vi "save parameters.vi"   [LabVIEW 2014]
uses:
  Start all VIs Globals.vi
  TIRF Lock/autofocus-globals.vi
  <vilib>/Utility/config.llb/Write Key (Boolean).vi
  <vilib>/Utility/config.llb/Write Key (Double).vi
  <vilib>/Utility/config.llb/Write Key (I32).vi
  <vilib>/Utility/config.llb/Write Key (U32).vi
  <vilib>/Utility/config.llb/NI_LVConfig.lvlib
types:
  T1 = enum32{"Invalid", "Standard", "Closed", "Hidden", "Minimized", "Maximized"}
  T2 = typedef "NI_LVConfig.lvlib/Config Data RefNum.ctl" = refnum<k1>
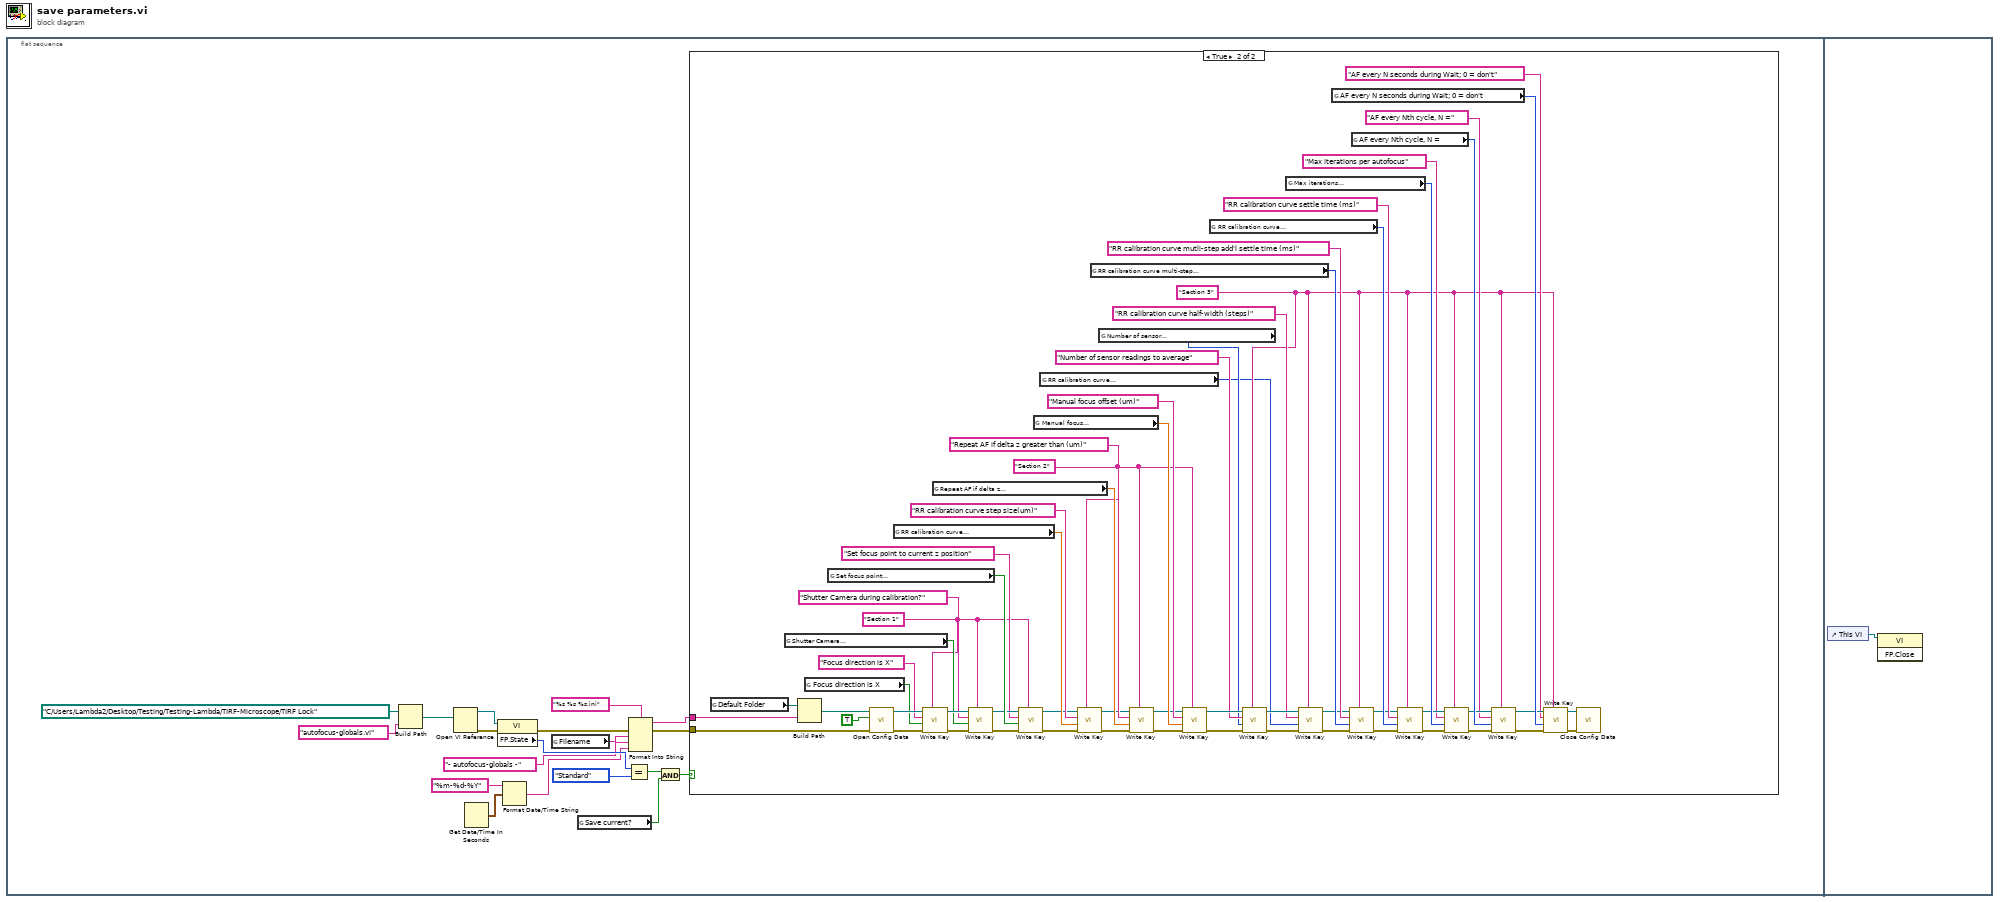
[diagram p0: block diagram]
diagram:
  n1 = flat-sequence {
    frame #0 {
      n2 = Build Path(base path=path "C:/Users/Lambda2/Desktop/Testing/Testing-Lambda/TIRF-Microscope/TIRF Lock", name or relative path="autofocus-globals.vi") -> (appended path=w18:path)
      n3 = Open VI Reference(vi path=w18) -> (vi reference=w17:refnum<vi>, error out=w16:errorcluster)  [unwired: 1 in, 4 out]
      n4 = Get Date/Time In Seconds() -> (seconds since 1Jan1904=w1:timestamp)
      n5 = property class="VI"(reference=w17, error in=w16) -> (error out=w7:errorcluster, "FP.State"=w13:T1)  [unwired: 1 out]
      n6 = Format Date/Time String(time format string (%c)="%m-%d-%Y", seconds (now)=w1) -> (date/time string=w3:string)  [unwired: 1 in]
      n7 = global read "Start all VIs Globals.vi" "Filename"() -> (w4:string)
      n8 = global read "Start all VIs Globals.vi" "Save current?"() -> (w10:bool)
      n9 = Equal?(x=w13, y=T1."Standard") -> (x = y?=w12:bool)
      n10 = Format Into String(format string="%s %s %s.ini", error in=w7, w4, "- autofocus-globals -", w3) -> (resulting string=w8:string, error out=w6:errorcluster)  [unwired: 1 in]
      n11 = And(x=w12, y=w10) -> (x .and. y?=w11:bool)
      n12 = case shown="True" w11 {
        tunnel: w6 -> [_ w32]
        tunnel: w8 -> [_ w34]
        frame False {
        }
        frame True {
          w22 = "Section 3"
          w38 = "Section 2"
          w39 = "Section 1"
          n13 = global read "Start all VIs Globals.vi" "Default Folder"() -> (w35:path)
          n14 = global read "autofocus-globals.vi" "Shutter Camera\nduring calibration?"() -> (w72:bool)
          n15 = Build Path(base path=w35, name or relative path=w34) -> (appended path=w33:path)
          n16 = global read "autofocus-globals.vi" "Focus direction is X"() -> (w78:bool)
          n17 = global read "autofocus-globals.vi" "Set focus point\nto current z position"() -> (w71:bool)
          n18 = call <vilib>:"Open Config Data.vi"("error in (no error)"=w32, "create file if necessary (T)"=TRUE, "configuration file path"=w33) -> ("error out"=w80:errorcluster, "refnum"=w79:T2)  [unwired: 7 out]
          n19 = global read "autofocus-globals.vi" "RR calibration curve\nstep size (um)"() -> (w68:ext)
          n20 = call-poly <vilib>:"Write Key.vi"("section"=w39, "error in (no error)"=w80, "value"=w78, "key"="Focus direction is X", "refnum"=w79) -> ("error out"=w76:errorcluster, "refnum out"=w74:T2)  [unwired: 5 out]
          n21 = global read "autofocus-globals.vi" "Repeat AF if delta z \ngreater than (um)"() -> (w66:dbl)
          n22 = call-poly <vilib>:"Write Key.vi"("section"=w39, "error in (no error)"=w76, "value"=w72, "key"="Shutter Camera during calibration?", "refnum"=w74) -> ("error out"=w75:errorcluster, "refnum out"=w70:T2)  [unwired: 5 out]
          n23 = call-poly <vilib>:"Write Key.vi"("section"=w39, "error in (no error)"=w75, "value"=w71, "key"="Set focus point to current z position", "refnum"=w70) -> ("error out"=w67:errorcluster, "refnum out"=w59:T2)  [unwired: 5 out]
          n24 = global read "autofocus-globals.vi" "Manual focus\noffset (um)"() -> (w65:dbl)
          n25 = global read "autofocus-globals.vi" "RR calibration curve\nhalf-width  (steps)"() -> (w20:u32)
          n26 = call-poly <vilib>:"Write Key.vi"("section"=w38, "error in (no error)"=w67, "value"=w68, "key"="RR calibration curve step size(um)", "refnum"=w59) -> ("error out"=w64:errorcluster, "refnum out"=w58:T2)  [unwired: 3 in, 2 out]
          n27 = global read "autofocus-globals.vi" "RR calibration curve multi-step\nadd'l settle time (ms)"() -> (w26:u16)
          n28 = global read "autofocus-globals.vi" "Number of sensor\nreadings to average"() -> (w21:i32)
          n29 = call-poly <vilib>:"Write Key.vi"("section"=w38, "error in (no error)"=w64, "value"=w66, "key"="Repeat AF if delta z greater than (um)", "refnum"=w58) -> ("error out"=w63:errorcluster, "refnum out"=w57:T2)  [unwired: 3 in, 2 out]
          n30 = call-poly <vilib>:"Write Key.vi"("section"=w38, "error in (no error)"=w63, "value"=w65, "key"="Manual focus offset (um)", "refnum"=w57) -> ("error out"=w56:errorcluster, "refnum out"=w55:T2)  [unwired: 3 in, 2 out]
          n31 = global read "autofocus-globals.vi" "RR calibration curve\nsettle time (ms)"() -> (w31:u32)
          n32 = call-poly <vilib>:"Write Key.vi"("section"=w22, "error in (no error)"=w56, "value"=w21, "key"="Number of sensor readings to average", "refnum"=w55) -> ("error out"=w54:errorcluster, "refnum out"=w46:T2)  [unwired: 4 in, 1 out]
          n33 = global read "autofocus-globals.vi" "Max iterations \nper autofocus"() -> (w51:i32)
          n34 = call-poly <vilib>:"Write Key.vi"("section"=w22, "error in (no error)"=w54, "value"=w20, "key"="RR calibration curve half-width (steps)", "refnum"=w46) -> ("error out"=w28:errorcluster, "refnum out"=w24:T2)  [unwired: 4 in, 1 out]
          n35 = global read "autofocus-globals.vi" "AF every N seconds during Wait; 0 = don't"() -> (w49:u32)
          n36 = call-poly <vilib>:"Write Key.vi"("section"=w22, "error in (no error)"=w28, "value"=w26, "key"="RR calibration curve mutli-step add'l settle time (ms)", "refnum"=w24) -> ("error out"=w27:errorcluster, "refnum out"=w23:T2)  [unwired: 4 in, 1 out]
          n37 = global read "autofocus-globals.vi" "AF every Nth cycle, N ="() -> (w50:u32)
          n38 = call-poly <vilib>:"Write Key.vi"("section"=w22, "error in (no error)"=w27, "value"=w31, "key"="RR calibration curve settle time (ms)", "refnum"=w23) -> ("error out"=w53:errorcluster, "refnum out"=w45:T2)  [unwired: 4 in, 1 out]
          n39 = call-poly <vilib>:"Write Key.vi"("section"=w22, "error in (no error)"=w53, "value"=w51, "key"="Max iterations per autofocus", "refnum"=w45) -> ("error out"=w52:errorcluster, "refnum out"=w44:T2)  [unwired: 4 in, 1 out]
          n40 = call-poly <vilib>:"Write Key.vi"("section"=w22, "error in (no error)"=w52, "value"=w50, "key"="AF every Nth cycle, N =", "refnum"=w44) -> ("error out"=w48:errorcluster, "refnum out"=w43:T2)  [unwired: 4 in, 1 out]
          n41 = call-poly <vilib>:"Write Key.vi"("section"=w22, "error in (no error)"=w48, "value"=w49, "key"="AF every N seconds during Wait; 0 = don't", "refnum"=w43) -> ("error out"=w37:errorcluster, "refnum out"=w36:T2)  [unwired: 4 in, 1 out]
          n42 = call <vilib>:"Close Config Data.vi"("error in (no error)"=w37, "refnum"=w36) -> ()  [unwired: 1 in, 9 out]
        }
      }
    }
    frame #1 {
      n43 = control-ref of="This VI"() -> (w82:refnum<vi>)
      n44 = invoke class="VI" method="FP.Close"(reference=w82) -> ()  [unwired: 2 in, 3 out]
    }
  }
